vi "Set_MultiVar_Values.vi"(8 "error in (no error)":errorcluster, 9 "varValues":dbl[](array[numeric]) format="%#_13g", 10 "varNames":string[](array[string]), 11 "mupExpr in":refnum<data-value>) -> (0 "error out":errorcluster, 3 "mupExpr out":refnum<data-value>)   [LabVIEW 2015, in "mupExpr.lvclass"]
uses:
  mupExpr.lvclass
  mupExpr.lvclass/mupExpr.ctl
  mupLib/mupSetVarValue.vi
  <vilib>/Utility/error.llb/Error Cluster From Error Code.vi
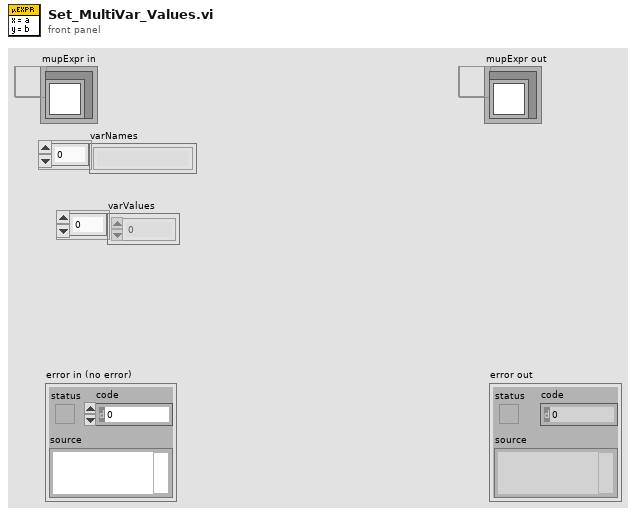
[diagram p1: front panel]
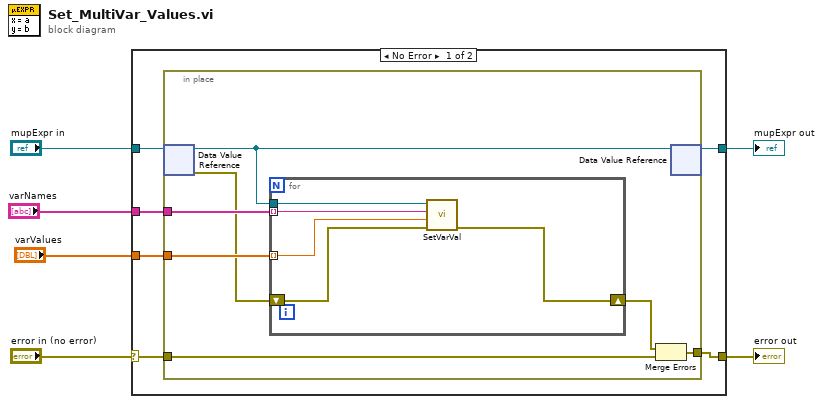
[diagram p0: block diagram]
diagram:
  n1 = case shown="No Error" "error in (no error)" {
    selector: "error in (no error)" -> [w7 w25]
    tunnel: "varValues" -> [w12 _]
    tunnel: "varNames" -> [w11 _]
    tunnel: "mupExpr in" -> [w10 w26]
    tunnel: [w9 w25] -> w3
    tunnel: [w8 w26] -> w2
    frame No Error {
      n2 = in-place {
        in-place-border: w7 -> [w15]
        in-place-border: w12 -> [w19]
        in-place-border: w11 -> [w18]
        in-place-border: [w14] -> w9
        n3 = in-place-dvr #1(w10) -> (w13:refnum<class "mupExpr.lvclass">, w17:errorcluster)
        n4 = for {
          tunnel: w18 -> [w24] mode=indexing
          tunnel: w19 -> [w23] mode=indexing
          shift-right: [w21] -> w16
          shift-left: w17 -> [w22]
          tunnel: w13 -> [w20]
          n5 = call "SetVarVal.vi"("error in (no error)"=w22, "varValue"=w23, "varName"=w24, "muExpr in"=w20) -> ("error out"=w21:errorcluster)  [unwired: 6 in, 1 out]
        }
        n6 = Merge Errors(w16, w15) -> (w14:errorcluster)
        n7 = in-place-dvr #1(w13) -> (w8:refnum<data-value>)  [unwired: 1 out]
      }
    }
    frame Error {
    }
  }
  "error out" <- w3
  "mupExpr out" <- w2
